vi "Update Camera Path.vi"(11 "Scene in":refnum<class "Scene.lvclass">) -> (3 "Scene out":refnum<class "Scene.lvclass">)   [LabVIEW 2020, in "Application.lvlib" / "Scene.lvclass"]
uses:
  Scene.lvclass
  Camera Movement.ctl
panel:
  in  "Left Speed":sgl
  in  "Fordward Speed":sgl=0.1
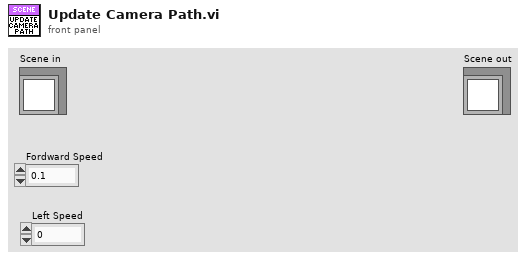
[diagram p1: front panel]
types:
  T1 = typedef "Application.lvlib/Scene.lvclass/Camera Movement.ctl" = enum16{"Forward", "Backwards", "Up", "Down", "Left", "Right", "Yaw CCW", "Yaw CW"}
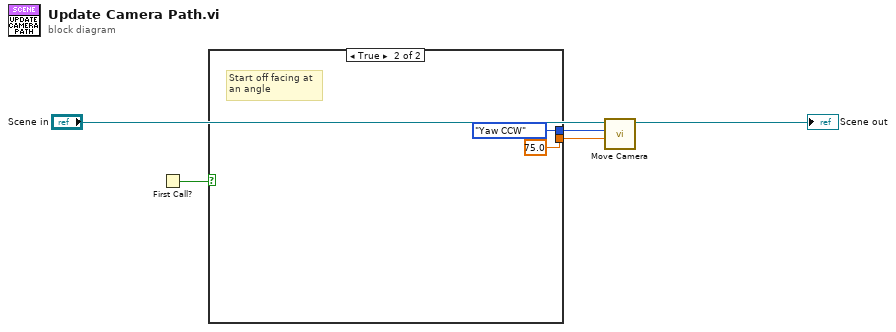
[diagram p0: block diagram]
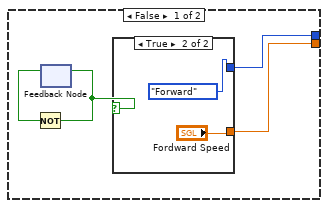
[diagram p2: hidden frame]
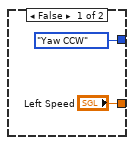
[diagram p3: hidden frame]
diagram:
  n1 = First Call?() -> (First Call?: T/F=w1:bool)
  n2 = case shown="True" w1 {
    tunnel: [w7 sgl 75.0 ("Fordward Speed")] -> w3
    tunnel: [w6 Camera_Movement."Yaw CCW" ("Camera Movement")] -> w2
    frame False {
      n3 = feedback #1() -> (w9:bool)  [unwired: 1 in]
      n4 = Not(x=w9) -> (.not. x?=w8:bool)
      n5 = feedback-in #1(w8) -> ()
      n6 = case shown="True" w8 {
        tunnel: ["Left Speed" "Fordward Speed"] -> w7
        tunnel: [Camera_Movement."Yaw CCW" ("Camera Movement") Camera_Movement."Forward" ("Camera Movement")] -> w6
        frame False {
        }
        frame True {
        }
      }
    }
    frame True {
      # "Start off facing at an angle"
    }
  }
  n7 = call "Move Camera.vi"("Camera Speed"=w3, "Camera Movement"=w2, "Scene in"="Scene in") -> ("Scene out"=→"Scene out":refnum<class "Scene.lvclass">)  [unwired: 8 in]
